vi "StartUp Sequence Open Loop Rev 1.3 - Not-As Retarded Engine Ramp Up.vi"() -> ()   [LabVIEW 2017]
panel:
  in  "Shut Off":bool
  out "ECU COM Port Out":refnum<visa-resource-name>
  out "Throttle Position":string
  out "Turbine RPM":string
  out "Turbine Temp":string
  out "Pump Voltage":string
  out "Error Out":errorcluster
  in  "Error In":errorcluster
  in  "ECU COM Port":refnum<visa-resource-name>
  out "Turbine State":string
  in  "Strt Sqnc":bool
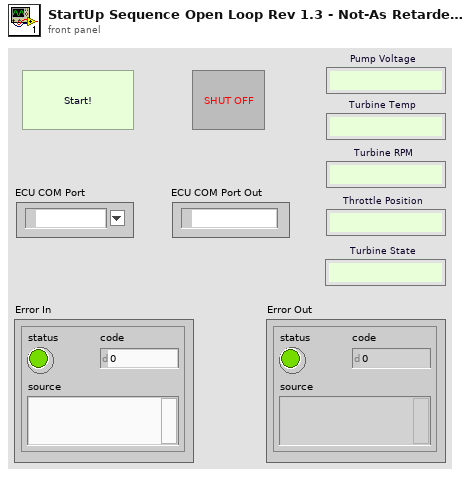
[diagram p1: front panel]
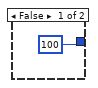
[diagram p2: hidden frame]
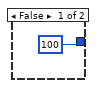
[diagram p3: hidden frame]
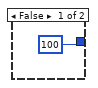
[diagram p4: hidden frame]
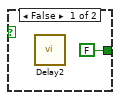
[diagram p6: hidden frame]
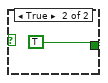
[diagram p7: hidden frame]
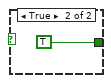
[diagram p8: hidden frame]
diagram:
  # "Disengage Starter Motor"
  # "Starter Motor 55%"
  # "Start button is inside a while loop that doesn't progess until True"
  # "Fuel Pump Mode 2"
  # "Fuel Pump to \nIdleRPMRate\n\"MODE 3\"???"
  # "BurnerValveOff"
  # "StarterMotorOff"
  # "GlowPlugOff"
  # "Start Up\nFuelPumpMode 1"
  # "BurnerValveIgnitionPercent"
  # "If False, each Case structure is set\nto an arbitrary Delay time of 0.2 s"
  # "Each Stage is inside a while loop so that \nthe sequence doesn't progress until True"
  n1 = while {
    tunnel: "Error In" -> [w131]
    tunnel: [w131] -> w23
    stop <- "Strt Sqnc" stop-if-true
  }
  n2 = while {
    tunnel: ["Shut Off"] -> w107
    tunnel: "ECU COM Port" -> [w133]
    stop <- "Shut Off" stop-if-true
    # "Turns off each individual component"
    n3 = case shown="True" "Shut Off" {
      tunnel: w133 -> [_ w137]
      frame False {
      }
      frame True {
        n4 = call "Delay11"() -> ("error out"=w135:errorcluster)  [unwired: 11 in]
        n5 = VISA Write(VISA resource name=w137, write buffer="SMD0", error in (no error)=w135) -> (VISA resource name out=w142:refnum<visa-resource-name>, error out=w155:errorcluster)  [unwired: 1 out]
        n6 = call "Delay6"("error in (no error)"=w155) -> ("error out"=w149:errorcluster)  [unwired: 10 in]
        n7 = VISA Write(VISA resource name=w142, write buffer="GPD0", error in (no error)=w149) -> (VISA resource name out=w140:refnum<visa-resource-name>, error out=w153:errorcluster)  [unwired: 1 out]
        n8 = call "Delay7"("error in (no error)"=w153) -> ("error out"=w148:errorcluster)  [unwired: 10 in]
        n9 = VISA Write(VISA resource name=w140, write buffer="FPM0", error in (no error)=w148) -> (VISA resource name out=w139:refnum<visa-resource-name>, error out=w152:errorcluster)  [unwired: 1 out]
        n10 = call "Delay8"("error in (no error)"=w152) -> ("error out"=w147:errorcluster)  [unwired: 10 in]
        n11 = VISA Write(VISA resource name=w139, write buffer="BVP0", error in (no error)=w147) -> (VISA resource name out=w138:refnum<visa-resource-name>, error out=w151:errorcluster)  [unwired: 1 out]
        n12 = call "Delay9"("error in (no error)"=w151) -> ("error out"=w146:errorcluster)  [unwired: 10 in]
        n13 = VISA Write(VISA resource name=w138, write buffer="FVP0", error in (no error)=w146) -> (error out=w150:errorcluster)  [unwired: 2 out]
        n14 = call "Delay10"("error in (no error)"=w150) -> ("error out"=w136:errorcluster)  [unwired: 10 in]
        n15 = flat-sequence {
          tunnel: w136 -> [w156]
          tunnel: [w156] -> _
          frame #0 {
            n16 = local write "Strt Sqnc"(FALSE ("Strt Sqnc")) -> ()
          }
        }
      }
    }
  }
  n17 = call "Initialize Com Port.vi"("Error In"=w23, "ECU COM Port"="ECU COM Port") -> ("Error Out"=w97:errorcluster, "ECU COM Port Out"=w22:refnum<visa-resource-name>)  [unwired: 8 in]
  n18 = while {
    tunnel: w23 -> [w163]
    tunnel: w22 -> [w162]
    stop <- w159 continue-if-true
    n19 = call "Get Engine Update.vi"("Error In"=w163, "ECU COM Port"=w162) -> ("Temperature"=w160:string, "RPMs"=w161:string)  [unwired: 6 in, 2 out]
    "Turbine RPM" <- w161
    "Turbine Temp" <- w160
    n20 = call "Safety Check.vi"("Temperature"=w160, "RPMs"=w161) -> ("Safe?"=w159:bool)  [unwired: 9 in]
    n21 = Not(x=w159) -> (.not. x?=w158:bool)
    n22 = Stop(stop? (T)=w158) -> ()
  }
  n23 = call "Set Glow Plug Duty Cycle.vi"("Error In"=w97, "Duty Cycle"=6, "ECU COM Port"=w22) -> ("Error Out"=w96:errorcluster, "ECU COM Port Out"=w93:refnum<visa-resource-name>)  [unwired: 7 in]
  n24 = flat-sequence {
    tunnel: w23 -> [_]
    frame #0 {
      n25 = local write "Turbine State"("Initializing Motor") -> ()
    }
  }
  n26 = call "Delay"("error in (no error)"=w96) -> ("error out"=w95:errorcluster)  [unwired: 10 in]
  n27 = call "Set Glow Plug Duty Cycle.vi"("Error In"=w95, "Duty Cycle"=19, "ECU COM Port"=w93) -> ("Error Out"=w94:errorcluster, "ECU COM Port Out"=w89:refnum<visa-resource-name>)  [unwired: 7 in]
  n28 = call "Delay"("error in (no error)"=w94) -> ("error out"=w90:errorcluster)  [unwired: 10 in]
  n29 = call "Set Starter Motor Duty Cycle.vi"("Error In"=w90, "Duty Cycle"=6, "ECU COM Port"=w89) -> ("Error Out"=w88:errorcluster, "ECU COM Port Out"=w86:refnum<visa-resource-name>)  [unwired: 7 in]
  n30 = call "Set Glow Plug Duty Cycle.vi"("Error In"=w88, "Duty Cycle"=15, "ECU COM Port"=w86) -> ("Error Out"=w87:errorcluster, "ECU COM Port Out"=w82:refnum<visa-resource-name>)  [unwired: 7 in]
  n31 = call "Delay"("error in (no error)"=w87) -> ("error out"=w84:errorcluster)  [unwired: 10 in]
  n32 = call "Set Starter Motor Duty Cycle.vi"("Error In"=w84, "Duty Cycle"=4, "ECU COM Port"=w82) -> ("Error Out"=w83:errorcluster, "ECU COM Port Out"=w81:refnum<visa-resource-name>)  [unwired: 7 in]
  n33 = call "Delay"("error in (no error)"=w83) -> ("error out"=w108:errorcluster)  [unwired: 10 in]
  n34 = while {
    tunnel: w108 -> [w167]
    tunnel: w81 -> [w166]
    tunnel: [w166] -> w118
    tunnel: [w167] -> w117
    stop <- w170 stop-if-true
    n35 = local read "Turbine RPM"() -> (w165:string)
    n36 = Decimal String To Number(string=w165) -> (number=w169:i32)  [unwired: 2 in, 1 out]
    n37 = Greater Or Equal?(x=w169, y=3300) -> (x >= y?=w171:bool)
    n38 = case shown="True" w171 {
      tunnel: [FALSE TRUE] -> w170
      frame False {
        n39 = call "Delay2"() -> ()  [unwired: 11 in, 1 out]
      }
      frame True {
      }
    }
  }
  n40 = flat-sequence {
    tunnel: w108 -> [_]
    frame #0 {
      n41 = local write "Turbine State"("Stage1 Check RPM") -> ()
    }
  }
  n42 = Stop(stop? (T)=w107) -> ()
  n43 = call "CmdSeparator7"("error in (no error)"=w117) -> ("error out"=w116:errorcluster)  [unwired: 10 in]
  n44 = VISA Write(VISA resource name=w118, write buffer="FPM160,016", error in (no error)=w116) -> (VISA resource name out=w69:refnum<visa-resource-name>, error out=w129:errorcluster)  [unwired: 1 out]
  n45 = call "CmdSeparator2"("error in (no error)"=w129) -> ("error out"=w80:errorcluster)  [unwired: 10 in]
  n46 = call "Set Burner Valve Percent.vi"("Error In"=w80, "Percent"=10, "ECU COM Port"=w69) -> ("Error Out"=w79:errorcluster, "ECU COM Port Out"=w68:refnum<visa-resource-name>)  [unwired: 7 in]
  n47 = call "CmdSeparator"("error in (no error)"=w79) -> ("error out"=w78:errorcluster)  [unwired: 10 in]
  n48 = call "Set Burner Valve Percent.vi"("Error In"=w78, "Percent"=31, "ECU COM Port"=w68) -> ("Error Out"=w77:errorcluster, "ECU COM Port Out"=w67:refnum<visa-resource-name>)  [unwired: 7 in]
  n49 = call "CmdSeparator10"("error in (no error)"=w77) -> ("error out"=w76:errorcluster)  [unwired: 10 in]
  n50 = call "Set Burner Valve Percent.vi"("Error In"=w76, "Percent"=35, "ECU COM Port"=w67) -> ("Error Out"=w75:errorcluster, "ECU COM Port Out"=w66:refnum<visa-resource-name>)  [unwired: 7 in]
  n51 = call "CmdSeparator11"("error in (no error)"=w75) -> ("error out"=w74:errorcluster)  [unwired: 10 in]
  n52 = call "Set Burner Valve Percent.vi"("Error In"=w74, "Percent"=39, "ECU COM Port"=w66) -> ("Error Out"=w73:errorcluster, "ECU COM Port Out"=w65:refnum<visa-resource-name>)  [unwired: 7 in]
  n53 = call "CmdSeparator12"("error in (no error)"=w73) -> ("error out"=w72:errorcluster)  [unwired: 10 in]
  n54 = call "Set Burner Valve Percent.vi"("Error In"=w72, "Percent"=43, "ECU COM Port"=w65) -> ("Error Out"=w71:errorcluster, "ECU COM Port Out"=w64:refnum<visa-resource-name>)  [unwired: 7 in]
  n55 = call "CmdSeparator13"("error in (no error)"=w71) -> ("error out"=w70:errorcluster)  [unwired: 10 in]
  n56 = call "Set Burner Valve Percent.vi"("Error In"=w70, "Percent"=47, "ECU COM Port"=w64) -> ("Error Out"=w43:errorcluster, "ECU COM Port Out"=w42:refnum<visa-resource-name>)  [unwired: 7 in]
  n57 = call "CmdSeparator6"("error in (no error)"=w43) -> ("error out"=w45:errorcluster)  [unwired: 10 in]
  n58 = call "Set Burner Valve Percent.vi"("Error In"=w45, "Percent"=51, "ECU COM Port"=w42) -> ("Error Out"=w38:errorcluster, "ECU COM Port Out"=w39:refnum<visa-resource-name>)  [unwired: 7 in]
  n59 = call "CmdSeparator8"("error in (no error)"=w38) -> ("error out"=w41:errorcluster)  [unwired: 10 in]
  n60 = call "Set Burner Valve Percent.vi"("Error In"=w41, "Percent"=55, "ECU COM Port"=w39) -> ("Error Out"=w34:errorcluster, "ECU COM Port Out"=w35:refnum<visa-resource-name>)  [unwired: 7 in]
  n61 = call "CmdSeparator14"("error in (no error)"=w34) -> ("error out"=w37:errorcluster)  [unwired: 10 in]
  n62 = call "Set Burner Valve Percent.vi"("Error In"=w37, "Percent"=59, "ECU COM Port"=w35) -> ("Error Out"=w33:errorcluster, "ECU COM Port Out"=w32:refnum<visa-resource-name>)  [unwired: 7 in]
  n63 = call "CmdSeparator9"("error in (no error)"=w33) -> ("error out"=w106:errorcluster)  [unwired: 10 in]
  n64 = flat-sequence {
    tunnel: w106 -> [_]
    frame #0 {
      n65 = local write "Turbine State"("Stage2 Check Temp.") -> ()
    }
  }
  n66 = while {
    tunnel: w32 -> [w177]
    tunnel: w106 -> [w178]
    tunnel: [w177] -> w53
    tunnel: [w178] -> w54
    stop <- w181 stop-if-true
    # "Stage2Temp(C)"
    n67 = local read "Turbine Temp"() -> (w176:string)
    n68 = Decimal String To Number(string=w176) -> (number=w179:i32)  [unwired: 2 in, 1 out]
    n69 = Greater Or Equal?(x=w179, y=90) -> (x >= y?=w182:bool)
    n70 = case shown="False" w182 {
      tunnel: [FALSE TRUE] -> w181
      frame False {
        n71 = call "Delay3"() -> ()  [unwired: 11 in, 1 out]
      }
      frame True {
      }
    }
  }
  n72 = call "Set Glow Plug Duty Cycle.vi"("Error In"=w54, "Duty Cycle"=0, "ECU COM Port"=w53) -> ("Error Out"=w52:errorcluster, "ECU COM Port Out"=w50:refnum<visa-resource-name>)  [unwired: 7 in]
  n73 = call "CmdSeparator3"("error in (no error)"=w52) -> ("error out"=w51:errorcluster)  [unwired: 10 in]
  n74 = VISA Write(VISA resource name=w50, write buffer="FPM160,021", error in (no error)=w51) -> (VISA resource name out=w47:refnum<visa-resource-name>, error out=w49:errorcluster)  [unwired: 1 out]
  n75 = call "Set Burner Valve Percent.vi"("Error In"=w49, "Percent"=80, "ECU COM Port"=w47) -> ("Error Out"=w31:errorcluster, "ECU COM Port Out"=w46:refnum<visa-resource-name>)  [unwired: 7 in]
  n76 = call "CmdSeparator18"("error in (no error)"=w31) -> ("error out"=w30:errorcluster)  [unwired: 10 in]
  n77 = call "Set Fuel Valve Percent.vi"("Error In"=w30, "Percent"=12, "ECU COM Port"=w46) -> ("Error Out"=w29:errorcluster, "ECU COM Port Out"=w48:refnum<visa-resource-name>)  [unwired: 7 in]
  n78 = call "CmdSeparator16"("error in (no error)"=w29) -> ("error out"=w103:errorcluster)  [unwired: 10 in]
  n79 = for {
    N: 4 -> [_]
    tunnel: [w185] -> _
    tunnel: [w199] -> _
    tunnel: w48 -> [w191]
    tunnel: w103 -> [w192]
    shift-right: [w190] -> w25
    shift-left: 12 -> [w196]
    shift-right: [w187] -> _
    shift-left: 80 -> [w193]
    tunnel: [w199] -> w18 mode=indexing
    tunnel: [w185] -> w26 mode=indexing
    n80 = Less?(x=w196, y=100) -> (x < y?=w197:bool)
    n81 = Less?(x=w193, y=100) -> (x < y?=w194:bool)
    n82 = case shown="True" w194 {
      tunnel: w193 -> [_ w203]
      tunnel: [100 w201] -> w187
      frame False {
      }
      frame True {
        n83 = Add(x=w203, y=5) -> (x+y=w201:i32)
      }
    }
    n84 = case shown="True" w197 {
      tunnel: w196 -> [_ w207]
      tunnel: [100 w205] -> w190
      frame False {
      }
      frame True {
        n85 = Add(x=w207, y=6) -> (x+y=w205:i32)
      }
    }
    n86 = call "Set Fuel Valve Percent.vi"("Error In"=w192, "Percent"=w190, "ECU COM Port"=w191) -> ("Error Out"=w189:errorcluster, "ECU COM Port Out"=w186:refnum<visa-resource-name>)  [unwired: 7 in]
    n87 = call "Set Burner Valve Percent.vi"("Error In"=w189, "Percent"=w187, "ECU COM Port"=w186) -> ("Error Out"=w188:errorcluster, "ECU COM Port Out"=w185:refnum<visa-resource-name>)  [unwired: 7 in]
    n88 = call "CmdSeparator17"("error in (no error)"=w188) -> ("error out"=w199:errorcluster)  [unwired: 10 in]
  }
  n89 = flat-sequence {
    tunnel: w18 -> [_]
    frame #0 {
      n90 = local write "Turbine State"("Pump Ramp Up") -> ()
    }
  }
  n91 = for {
    N: 10 -> [_]
    tunnel: [w215] -> w2
    tunnel: [w226] -> w4
    shift-right: [w222] -> _
    shift-left: w25 -> [w223]
    tunnel: w18 -> [w219] mode=indexing
    tunnel: w26 -> [w218] mode=indexing
    shift-right: [w209] -> w20
    shift-left: 21 -> [w210]
    n92 = Less?(x=w223, y=100) -> (x < y?=w224:bool)
    n93 = Add(x=w210, y=1) -> (x+y=w209:i32)
    n94 = case shown="True" w224 {
      tunnel: w223 -> [_ w230]
      tunnel: [100 w228] -> w222
      frame False {
      }
      frame True {
        n95 = Add(x=w230, y=5) -> (x+y=w228:i32)
      }
    }
    n96 = call "Set Fuel Valve Percent.vi"("Error In"=w219, "Percent"=w222, "ECU COM Port"=w218) -> ("Error Out"=w221:errorcluster, "ECU COM Port Out"=w220:refnum<visa-resource-name>)  [unwired: 7 in]
    n97 = call "Set Burner Valve Percent.vi"("Error In"=w221, "Percent"=100 ("y"), "ECU COM Port"=w220) -> ("Error Out"=w213:errorcluster, "ECU COM Port Out"=w216:refnum<visa-resource-name>)  [unwired: 7 in]
    n98 = call "Set Pump Fow Rate.vi"("Error In"=w213, "Pulse Width"=w209, "Voltage"=160 ("y"), "ECU COM Port"=w216) -> ("Error Out"=w214:errorcluster, "ECU COM Port Out"=w215:refnum<visa-resource-name>)  [unwired: 6 in]
    n99 = call "CmdSeparator20"("error in (no error)"=w214) -> ("error out"=w226:errorcluster)  [unwired: 10 in]
  }
  n100 = call "Set Starter Motor Duty Cycle.vi"("Error In"=w4, "Duty Cycle"=11, "ECU COM Port"=w2) -> ("Error Out"=w5:errorcluster, "ECU COM Port Out"=w3:refnum<visa-resource-name>)  [unwired: 7 in]
  n101 = flat-sequence {
    tunnel: w4 -> [_]
    frame #0 {
      n102 = local write "Turbine State"("Secondary Pump Ramp Up") -> ()
    }
  }
  n103 = for {
    N: 3 -> [_]
    tunnel: [w240] -> w19
    tunnel: [w246] -> w17
    tunnel: [w232] -> _ mode=indexing
    tunnel: w3 -> [w243]
    shift-right: [w234] -> _
    shift-left: w20 -> [w235]
    tunnel: w5 -> [w232]
    n104 = Add(x=w235, y=10) -> (x+y=w234:i32)
    n105 = call "Set Fuel Valve Percent.vi"("Error In"=w232, "Percent"=100 ("y"), "ECU COM Port"=w243) -> ("Error Out"=w245:errorcluster, "ECU COM Port Out"=w244:refnum<visa-resource-name>)  [unwired: 7 in]
    n106 = call "Set Burner Valve Percent.vi"("Error In"=w245, "Percent"=0 ("y"), "ECU COM Port"=w244) -> ("Error Out"=w238:errorcluster, "ECU COM Port Out"=w241:refnum<visa-resource-name>)  [unwired: 7 in]
    n107 = call "Set Pump Fow Rate.vi"("Error In"=w238, "Pulse Width"=w234, "Voltage"=160 ("y"), "ECU COM Port"=w241) -> ("Error Out"=w239:errorcluster, "ECU COM Port Out"=w240:refnum<visa-resource-name>)  [unwired: 6 in]
    n108 = call "CmdSeparator15"("error in (no error)"=w239) -> ("error out"=w246:errorcluster)  [unwired: 10 in]
  }
  n109 = flat-sequence {
    tunnel: w17 -> [_]
    frame #0 {
      n110 = local write "Turbine State"("Hold on to your butts!") -> ()
    }
  }
  n111 = while {
    tunnel: w17 -> [w249]
    tunnel: w19 -> [w248]
    tunnel: [w249] -> w15
    tunnel: [w248] -> w16
    stop <- w250 stop-if-true
    n112 = local read "Turbine RPM"() -> (w253:string)
    n113 = Decimal String To Number(string=w253) -> (number=w252:i32)  [unwired: 2 in, 1 out]
    n114 = Greater?(x=w252, y=30000) -> (0:w250:bool)
  }
  n115 = call "Set Pump Fow Rate.vi"("Error In"=w15, "Pulse Width"=255 ("y"), "Voltage"=80 ("y"), "ECU COM Port"=w16) -> ("Error Out"=w12:errorcluster, "ECU COM Port Out"=w11:refnum<visa-resource-name>)  [unwired: 6 in]
  n116 = while {
    tunnel: w12 -> [w255]
    tunnel: w11 -> [w254]
    tunnel: [w255] -> w6
    tunnel: [w254] -> w9
    stop <- w256 stop-if-true
    n117 = local read "Turbine RPM"() -> (w259:string)
    n118 = Decimal String To Number(string=w259) -> (number=w258:i32)  [unwired: 2 in, 1 out]
    n119 = Greater?(x=w258, y=44000) -> (0:w256:bool)
  }
  n120 = call "Set Starter Motor Duty Cycle.vi"("Error In"=w6, "Duty Cycle"=0, "ECU COM Port"=w9) -> ("Error Out"=w10:errorcluster, "ECU COM Port Out"=w8:refnum<visa-resource-name>)  [unwired: 7 in]
  n121 = flat-sequence {
    tunnel: w6 -> [_]
    frame #0 {
      n122 = local write "Turbine State"("Acheived Idle RPM") -> ()
    }
  }
  n123 = VISA Write(VISA resource name=w8, write buffer="SMD0", error in (no error)=w10) -> (VISA resource name out=w124:refnum<visa-resource-name>, error out=w126:errorcluster)  [unwired: 1 out]
  n124 = call "CmdSeparator4"("error in (no error)"=w126) -> ("error out"=w125:errorcluster)  [unwired: 10 in]
  n125 = VISA Write(VISA resource name=w124, write buffer="BVV0", error in (no error)=w125) -> (VISA resource name out=w121:refnum<visa-resource-name>, error out=w120:errorcluster)  [unwired: 1 out]
  n126 = call "CmdSeparator5"("error in (no error)"=w120) -> ("error out"=w122:errorcluster)  [unwired: 10 in]
  n127 = VISA Write(VISA resource name=w121, write buffer="FPM3", error in (no error)=w122) -> (VISA resource name out=w119:refnum<visa-resource-name>, error out=w110:errorcluster)  [unwired: 1 out]
  n128 = while {
    tunnel: w119 -> [w267]
    tunnel: w110 -> [w266]
    tunnel: [w264] -> w109
    tunnel: [w263] -> w112
    stop <- w278 stop-if-true
    # "Idle RPM"
    n129 = VISA Write(VISA resource name=w267, write buffer="RQR", error in (no error)=w266) -> (VISA resource name out=w274:refnum<visa-resource-name>, error out=w276:errorcluster)  [unwired: 1 out]
    n130 = call "CmdDelay4"("error in (no error)"=w276) -> ("error out"=w275:errorcluster)  [unwired: 10 in]
    n131 = property class="Instr"(reference=w274, error in=w275) -> (reference out=w271:refnum<visa-resource-name>, error out=w272:errorcluster, "Bytes at Port"=w273:u32)
    n132 = VISA Read(VISA resource name=w271, byte count=w273, error in (no error)=w272) -> (VISA resource name out=w263:refnum<visa-resource-name>, read buffer=w265:string, error out=w264:errorcluster)  [unwired: 1 out]
    n133 = String Subset(string=w265, offset (0)=3) -> (substring=w269:string)  [unwired: 1 in]
    n134 = local write "Turbine RPM"(w265) -> ()
    n135 = Decimal String To Number(string=w269) -> (number=w268:i32)  [unwired: 2 in, 1 out]
    n136 = Greater Or Equal?(x=w268, y=44000) -> (x >= y?=w262:bool)
    n137 = case shown="False" w262 {
      tunnel: [FALSE TRUE] -> w278
      frame False {
        n138 = call "Delay5"() -> ()  [unwired: 11 in, 1 out]
      }
      frame True {
      }
    }
  }
  n139 = flat-sequence {
    tunnel: w110 -> [_]
    frame #0 {
      n140 = local write "Turbine State"("Stage4 Check Idle RPM") -> ()
    }
  }
  n141 = flat-sequence {
    tunnel: w109 -> [_]
    frame #0 {
      n142 = local write "Turbine State"("Stage5 Idle RPM Achieved") -> ()
    }
  }
  n143 = VISA Write(VISA resource name=w112, write buffer="END") -> (VISA resource name out=→"ECU COM Port Out":refnum<visa-resource-name>, error out=w105:errorcluster)  [unwired: 1 in, 1 out]
  n144 = flat-sequence {
    tunnel: w105 -> [w283]
    tunnel: [w283] -> w104
    frame #0 {
      n145 = local write "Strt Sqnc"(FALSE ("Strt Sqnc")) -> ()
    }
  }
  "Error Out" <- w104
